vi "DTM Transmitter Test.vi"() -> ()   [LabVIEW 2025, in "Nordic nRF52 DK DTM Test.lvlib"]
uses:
  Nordic nRF52 DK DTM Test.lvlib
  PacketType.ctl
  TxRx.ctl
  <vilib>/RFmx/BT/mx/RFmxBT.llb/RFmxBT Select Measurement (Single).vi
  <vilib>/RFmx/BT/mx/RFmxBT.llb/RFmxBT ModAcc Fetch df2max Trace.vi
  <vilib>/RFmx/BT/mx/RFmxBT.llb/RFmxBT ModAcc Fetch df2.vi
  <vilib>/RFmx/BT/mx/RFmxBT.llb/RFmxBT TXP Fetch Powers.vi
  <vilib>/RFmx/BT/mx/RFmxBT.llb/RFmxBT TXP Fetch Power Trace.vi
  <vilib>/RFmx/BT/mx/RFmxBT.llb/RFmxBT ACP Fetch Offset Measurement (Array).vi
  <vilib>/RFmx/BT/mx/RFmxBT.llb/RFmxBT ACP Fetch Absolute Power Trace.vi
  <vilib>/RFmx/BT/mx/RFmxBT.llb/RFmxBT ACP Fetch Mask Trace.vi
  <vilib>/RFmx/BT/mx/RFmxBT.llb/RFmxBT ACP Fetch Spectrum.vi
  Measurement.ctl
  <vilib>/RFmx/BT/mx/RFmxBT.llb/RFmxBT ModAcc Fetch df1max Trace.vi
  <vilib>/RFmx/BT/mx/RFmxBT.llb/RFmxBT ModAcc Fetch df1.vi
panel:
  in  "LE Data Rate (bps)":i32(ring)=1000000 items=["125K"=125000, "500K"=500000, "1M"=1000000, "2M"=2000000, "3M"=3000000, "4M"=4000000, "6M"=6000000, "7.5M"=7500000]
  in  "BLE Channel Number (0-39)":u8=19
  in  "Measurements":enum32{"ACLR", "Txp", "df1", "df2"}(tab)
  out "Offset Measurements":T1(array[cluster]) {"Upper Relative Power (dB)" format="%.2f"; "Lower Relative Power (dB)" format="%.2f"; "Upper Absolute Power (dBm)" format="%.2f"; "Lower Absolute Power (dBm)" format="%.2f"}
  out "ACP Trace":cluster{"x0":dbl, "dx":dbl, "y":sgl[]}[](graph)
  out "Average Power Minimum (dBm)":dbl format="%.2f"
  out "Average Power Maximum (dBm)":dbl format="%.2f"
  out "Average Power Mean (dBm)":dbl format="%.2f"
  out "Power Trace":cluster{"x0":dbl, "dx":dbl, "y":sgl[]}(graph)
  out "df1max Trace":cluster{"X":sgl, "Y":sgl}[](graph)
  out "df1avg  Minimum (Hz)":dbl format="%.3p"
  out "df1avg Maximum (Hz)":dbl format="%.3p"
  out "df2max Trace":cluster{"X":sgl, "Y":sgl}[](graph)
  out "% Symbols above Threshold":dbl format="%.3p"
  out "df2avg Minimum (Hz)":dbl format="%.3p"
  out "error out":errorcluster
  in  "External Attenuation":dbl=1.1
  in  "Frequency Reference Source":string(combo)="OnboardClock"
  in  "Resource Name":refnum<k15>="VST"
  in  "Com Port Resource":refnum<visa-resource-name>="COM3"
  in  "Baud Rate":u32=19200
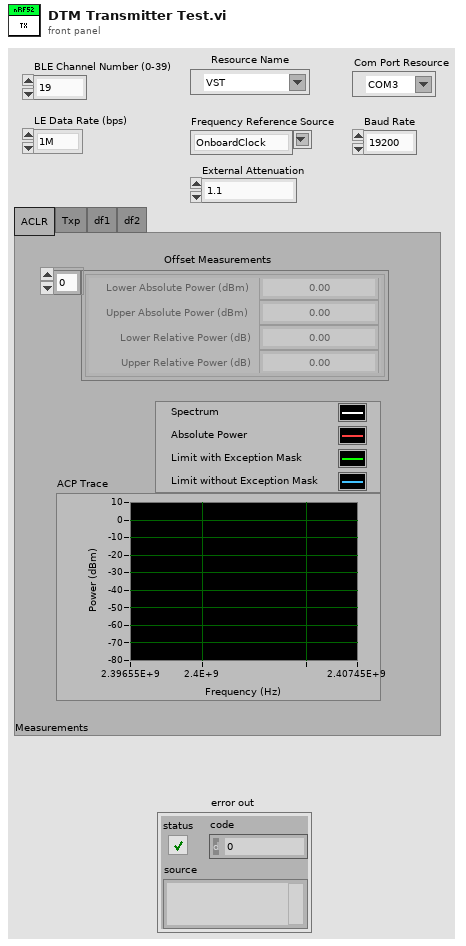
[diagram p1: front panel]
types:
  T1 = cluster{"Lower Absolute Power (dBm)":dbl, " Upper Absolute Power (dBm)":dbl, " Lower Relative Power (dB)":dbl, " Upper Relative Power (dB)":dbl}[]
  T2 = typedef "Nordic nRF52 DK DTM Test.lvlib/Measurement.ctl" = enum16{"Txp", "ACLR", "df1", "df2"}
  T3 = typedef "Nordic nRF52 DK DTM Test.lvlib/TxRx.ctl" = enum16{"Tx", "Rx"}
  T4 = typedef "niRFmx Instrument Handle.ctl" = refnum<k21>
  T5 = typedef "Nordic nRF52 DK DTM Test.lvlib/PacketType.ctl" = enum16{"PRBS9", "DF1", "DF2"}
  T6 = cluster{"Lower Absolute Power (dBm)":dbl, " Upper Absolute Power (dBm)":dbl, " Lower Relative Power (dB)":dbl, " Upper Relative Power (dB)":dbl}
  T7 = enum16{"TXP", "ModAcc", "20dBBandwidth", "FrequencyRange", "ACP", "PowerRamp", "ModSpectrum"}
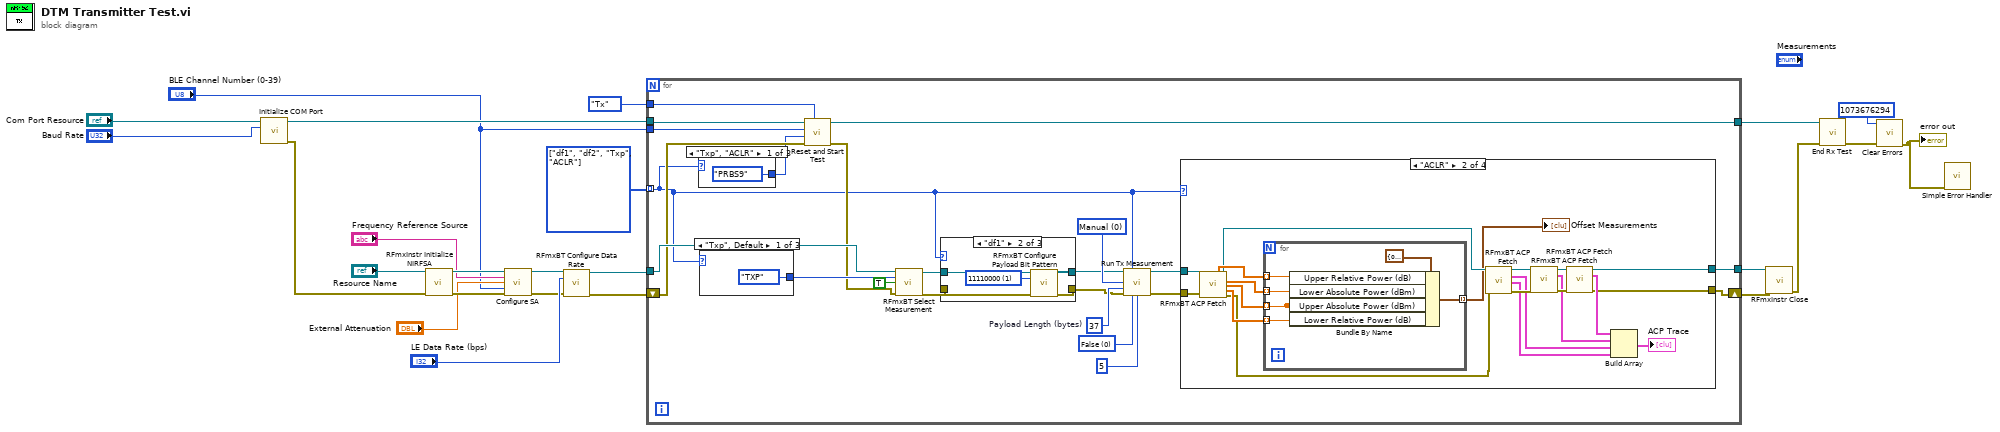
[diagram p0: block diagram]
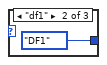
[diagram p2: hidden frame]
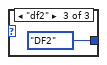
[diagram p3: hidden frame]
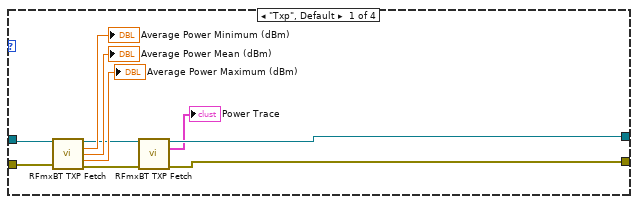
[diagram p4: hidden frame]
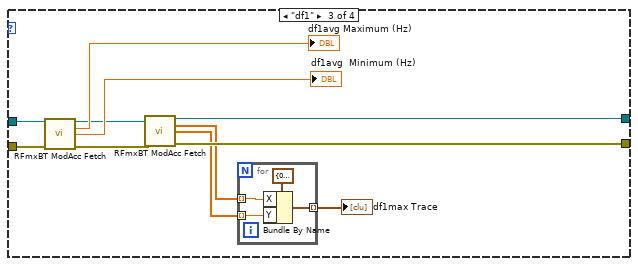
[diagram p5: hidden frame]
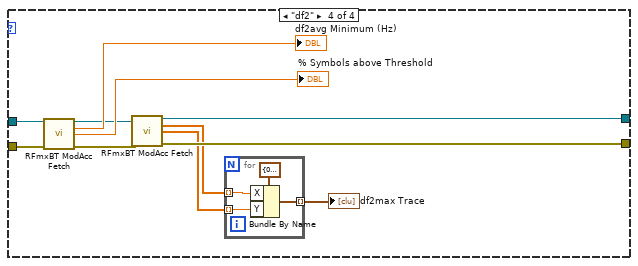
[diagram p6: hidden frame]
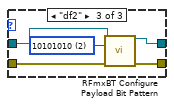
[diagram p8: hidden frame]
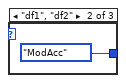
[diagram p9: hidden frame]
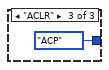
[diagram p10: hidden frame]
diagram:
  w10 = T2[] [enum."df1", enum."df2", enum."Txp", enum."ACLR"] items=["Txp", "ACLR", "df1", "df2"] ("Measurements")
  n1 = call "Initialize COM Port.vi"("baud rate (9600)"="Baud Rate", "VISA Refnum in"="Com Port Resource") -> ("error out"=w9:errorcluster, "VISA Refnum out"=w8:refnum<visa-resource-name>)  [unwired: 8 in]
  n2 = call <vilib>:"RFmxInstr Initialize NIRFSA.vi"("Resource Name"="Resource Name", "error in (no error)"=w9) -> ("Instrument Handle Out"=w22:refnum<k21>, "error out"=w23:errorcluster)  [unwired: 11 in, 1 out]
  n3 = call "Configure SA.vi"("Refnum in"=w22, "Frequency Reference Source"="Frequency Reference Source", "External Attenuation"="External Attenuation", "BLE  Channel"="BLE Channel Number (0-39)", "error in (no error)"=w23) -> ("Refnum out"=w12:T4, "error out"=w14:errorcluster)  [unwired: 9 in]
  n4 = call <vilib>:"RFmxBT Configure Data Rate.vi"("Instrument Handle In"=w12, "Data Rate (bps)"="LE Data Rate (bps)", "error in (no error)"=w14) -> ("Instrument Handle Out"=w11:refnum<k21>, "error out"=w13:errorcluster)  [unwired: 11 in]
  n5 = for {
    tunnel: w11 -> [w39]
    shift-right: [w25] -> w16
    shift-left: w13 -> [w31]
    tunnel: [w40] -> w17
    tunnel: w10 -> [w26] mode=indexing
    tunnel: w8 -> [w33]
    tunnel: "BLE Channel Number (0-39)" -> [w32]
    tunnel: TxRx."Tx" ("Tx/Rx") -> [w29]
    tunnel: [w27] -> w4
    w44 = 0 items=["False", "True"] ("Averaging Enabled")
    w46 = 0 items=["Manual", "Auto"] ("Payload Length Mode")
    w45 = 37  # Payload Length (bytes)
    n6 = case shown="\"Txp\", \"ACLR\"" w26 {
      tunnel: [PacketType."PRBS9" ("Tx Packet Type") PacketType."DF1" ("Tx Packet Type") PacketType."DF2" ("Tx Packet Type")] -> w28
      frame "Txp", "ACLR" {
      }
      frame "df1" {
      }
      frame "df2" {
      }
    }
    n7 = case shown="\"Txp\", Default" w26 {
      tunnel: [T7."TXP" ("Measurement") T7."ModAcc" ("Measurement") T7."ACP" ("Measurement")] -> w38
      frame "Txp", Default {
      }
      frame "df1", "df2" {
      }
      frame "ACLR" {
      }
    }
    n8 = call "Reset and Start Test.vi"("Tx/Rx"=w29, "error in (no error)"=w31, "Tx Packet Type"=w28, "BLE Channel Number (0-39)"=w32, "VISA Refnum in"=w33) -> ("error out"=w30:errorcluster, "VISA Refnum out"=w27:refnum<visa-resource-name>)  [unwired: 4 in, 1 out]
    n9 = call-poly <vilib>:"RFmxBT Select Measurement.vi"("Instrument Handle In"=w39, "Measurement"=w38, "Enable All Traces"=TRUE, "error in (no error)"=w30) -> ("Instrument Handle Out"=w37:refnum<k21>, "error out"=w36:errorcluster)  [unwired: 10 in]
    n10 = case shown="\"df1\"" w26 {
      tunnel: [w118 w122 w126] -> w42
      tunnel: [w117 w121 w125] -> w41
      tunnel: w37 -> [w117 w120 w124]
      tunnel: w36 -> [w118 w119 w127]
      frame "Txp", "ACLR" {
      }
      frame "df1" {
        w123 = 1 items=["Standard Defined", "11110000", "10101010"] ("df1")
        n11 = call <vilib>:"RFmxBT Configure Payload Bit Pattern.vi"("Instrument Handle In"=w120, "Payload Bit Pattern"=w123, "error in (no error)"=w119) -> ("Instrument Handle Out"=w121:refnum<k21>, "error out"=w122:errorcluster)  [unwired: 11 in]
      }
      frame "df2" {
        w128 = 2 items=["Standard Defined", "11110000", "10101010"] ("df1")
        n12 = call <vilib>:"RFmxBT Configure Payload Bit Pattern.vi"("Instrument Handle In"=w124, "Payload Bit Pattern"=w128, "error in (no error)"=w127) -> ("Instrument Handle Out"=w125:refnum<k21>, "error out"=w126:errorcluster)  [unwired: 11 in]
      }
    }
    n13 = call "Run Tx Measurement.vi"("Refnum in"=w41, "Measurement"=w26, "Payload Length Mode"=w46, "Payload Length (bytes)"=w45, "error in (no error)"=w42, "Averaging Enabled"=w44, "Averaging Count"=5) -> ("Refnum out"=w47:T4, "error out"=w34:errorcluster)  [unwired: 7 in]
    n14 = case shown="\"ACLR\"" w26 {
      tunnel: w47 -> [w59 w76 w97 w112]
      tunnel: w34 -> [w60 w75 w94 w109]
      tunnel: [w52 w63 w90 w105] -> w25
      tunnel: [w53 w62 w87 w102] -> w40
      frame "Txp", Default {
        n15 = call-poly <vilib>:"RFmxBT TXP Fetch.vi"("Instrument Handle In"=w59, "error in (no error)"=w60) -> ("Instrument Handle Out"=w55:refnum<k21>, "Average Power Mean (dBm)"=→"Average Power Minimum (dBm)":dbl, "Average Power Maximum (dBm)"=→"Average Power Mean (dBm)":dbl, "Average Power Minimum (dBm)"=→"Average Power Maximum (dBm)":dbl, "error out"=w54:errorcluster)  [unwired: 8 in, 1 out]
        n16 = call-poly <vilib>:"RFmxBT TXP Fetch.vi"("Instrument Handle In"=w55, "error in (no error)"=w54) -> ("Instrument Handle Out"=w53:refnum<k21>, "Power (dBm)"=→"Power Trace":cluster{"x0":dbl, "dx":dbl, "y":sgl[]}, "error out"=w52:errorcluster)  [unwired: 11 in]
      }
      frame "ACLR" {
        n17 = call-poly <vilib>:"RFmxBT ACP Fetch.vi"("Instrument Handle In"=w76, "error in (no error)"=w75) -> ("Upper Relative Power (dB)"=w80:dbl[], "Instrument Handle Out"=w65:refnum<k21>, "Lower Absolute Power (dBm)"=w77:dbl[], "Upper Absolute Power (dBm)"=w78:dbl[], "Lower Relative Power (dB)"=w79:dbl[], "error out"=w64:errorcluster)  [unwired: 6 in, 2 out]
        n18 = for {
          tunnel: w77 -> [w86] mode=indexing
          tunnel: [w85] -> w61 mode=indexing
          tunnel: [w84] -> _ mode=indexing
          tunnel: w78 -> [w84] mode=indexing
          tunnel: w79 -> [w83] mode=indexing
          tunnel: w80 -> [w82] mode=indexing
          n19 = Bundle By Name(cluster=T6 {"Lower Absolute Power (dBm)"=0.0, " Upper Absolute Power (dBm)"=0.0, " Lower Relative Power (dB)"=0.0, " Upper Relative Power (dB)"=0.0} ("Offset Measurement"), "Upper Relative Power (dB)"=w82, "Lower Absolute Power (dBm)"=w86, "Upper Absolute Power (dBm)"=w84, "Lower Relative Power (dB)"=w83) -> (w85:T6)
        }
        "Offset Measurements" <- w61
        n20 = call-poly <vilib>:"RFmxBT ACP Fetch.vi"("Instrument Handle In"=w65, "error in (no error)"=w64) -> ("Instrument Handle Out"=w71:refnum<k21>, "Limit With Exception Mask"=w68:cluster{"x0":dbl, "dx":dbl, "y":sgl[]}, "Limit Without Exception Mask"=w67:cluster{"x0":dbl, "dx":dbl, "y":sgl[]}, "error out"=w72:errorcluster)  [unwired: 10 in]
        n21 = call-poly <vilib>:"RFmxBT ACP Fetch.vi"("Instrument Handle In"=w71, "error in (no error)"=w72) -> ("Instrument Handle Out"=w73:refnum<k21>, "Absolute Power"=w69:cluster{"x0":dbl, "dx":dbl, "y":sgl[]}, "error out"=w74:errorcluster)  [unwired: 11 in]
        n22 = call-poly <vilib>:"RFmxBT ACP Fetch.vi"("Instrument Handle In"=w73, "error in (no error)"=w74) -> ("Instrument Handle Out"=w62:refnum<k21>, "Spectrum"=w70:cluster{"x0":dbl, "dx":dbl, "y":sgl[]}, "error out"=w63:errorcluster)  [unwired: 11 in]
        n23 = Build Array(w70, w69, w68, w67) -> (→"ACP Trace":cluster{"x0":dbl, "dx":dbl, "y":sgl[]}[])
      }
      frame "df1" {
        n24 = call-poly <vilib>:"RFmxBT ModAcc Fetch.vi"("Instrument Handle In"=w97, "error in (no error)"=w94) -> ("Instrument Handle Out"=w91:refnum<k21>, "df1avg Maximum (Hz)"=→"df1avg Maximum (Hz)":dbl, "df1avg  Minimum (Hz)"=→"df1avg  Minimum (Hz)":dbl, "error out"=w92:errorcluster)  [unwired: 10 in]
        n25 = call-poly <vilib>:"RFmxBT ModAcc Fetch.vi"("Instrument Handle In"=w91, "error in (no error)"=w92) -> ("Instrument Handle Out"=w87:refnum<k21>, "Time (s)"=w89:sgl[], "df1max (Hz)"=w88:sgl[], "error out"=w90:errorcluster)  [unwired: 10 in]
        n26 = for {
          tunnel: [w100] -> w93 mode=indexing
          tunnel: w89 -> [w99] mode=indexing
          tunnel: w88 -> [w98] mode=indexing
          n27 = Bundle By Name(cluster=cluster{"X":sgl, "Y":sgl} {"X"=0.0, "Y"=0.0}, "X"=w99, "Y"=w98) -> (w100:cluster{"X":sgl, "Y":sgl})
        }
        "df1max Trace" <- w93
      }
      frame "df2" {
        n28 = call-poly <vilib>:"RFmxBT ModAcc Fetch.vi"("Instrument Handle In"=w112, "error in (no error)"=w109) -> ("Instrument Handle Out"=w106:refnum<k21>, "df2avg Minimum (Hz)"=→"df2avg Minimum (Hz)":dbl, "Percentage of Symbols above df2max Threshold (%)"=→"% Symbols above Threshold":dbl, "error out"=w107:errorcluster)  [unwired: 10 in]
        n29 = call-poly <vilib>:"RFmxBT ModAcc Fetch.vi"("Instrument Handle In"=w106, "error in (no error)"=w107) -> ("Instrument Handle Out"=w102:refnum<k21>, "Time (s)"=w104:sgl[], "df2max (Hz)"=w103:sgl[], "error out"=w105:errorcluster)  [unwired: 10 in]
        n30 = for {
          tunnel: [w115] -> w108 mode=indexing
          tunnel: w104 -> [w114] mode=indexing
          tunnel: w103 -> [w113] mode=indexing
          n31 = Bundle By Name(cluster=cluster{"X":sgl, "Y":sgl} {"X"=0.0, "Y"=0.0}, "X"=w114, "Y"=w113) -> (w115:cluster{"X":sgl, "Y":sgl})
        }
        "df2max Trace" <- w108
      }
    }
  }
  n32 = call <vilib>:"RFmxInstr Close.vi"("Instrument Handle In"=w17, "error in (no error)"=w16) -> ("error out"=w7:errorcluster)  [unwired: 13 in]
  n33 = call "End Rx Test.vi"("error in (no error)"=w7, "VISA Refnum in"=w4) -> ("error out"=w2:errorcluster)  [unwired: 7 in, 2 out]
  n34 = call <vilib>:"Clear Errors.vi"("error in (no error)"=w2, "specific error code to clear (0: all)"=1073676294) -> ("error out"=w1:errorcluster)  [unwired: 4 in, 1 out]
  "error out" <- w1
  n35 = call <vilib>:"Simple Error Handler.vi"("error in (no error)"=w1) -> ()  [unwired: 4 in, 5 out]
